vi "DCMotor_GetKrakenX44_FOC.vi"(11 "Num Motors":i32=1) -> (3 "DCMOTOR":T1 {"Jr_KgM2" format="%13.5p"; "L_H" format="%13.5p"; "Kt_NMPerAmp" format="%13.5p"; "KvINV_RadPerSecPerVolt" format="%13.5p"; "R_Ohms" format="%13.5p"; "FreeSpeed_RadPerSec" format="%13.5p"; "FreeCurrent_Amps" format="%13.5p"; "StallCurrent_Amps" format="%13.5p"; "StallTorque_NM" format="%13.5p"; "nominalVoltage_Volts" format="%13.5p"})   [LabVIEW 2019, in "Trajectory_Library.lvlib"]
doc: "Creates a new DC MOTOR data cluster with the specified values. for a set of Kraken X44 with FOC enabled motors. \n\nInputs: \n - Num Motors -- The number of motors used together in this sytem driving the same load.\n\nOutputs:\n - DCMOTOR -- Cluster containing the motor modeling constants for this set of motors."
uses:
  TypeDef/DCMOTOR.CTL
  Trajectory_Library.lvlib
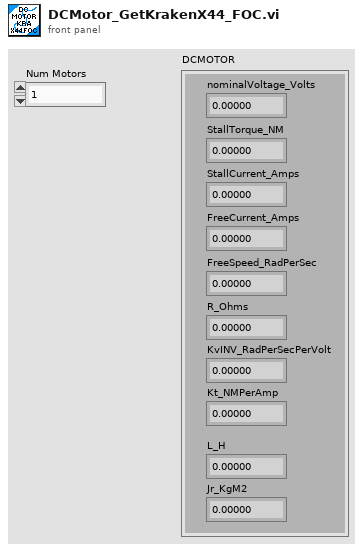
[diagram p1: front panel]
types:
  T1 = typedef "Trajectory_Library.lvlib/DCMOTOR.CTL" = cluster{"nominalVoltage_Volts":dbl, "StallTorque_NM":dbl, "StallCurrent_Amps":dbl, "FreeCurrent_Amps":dbl, "FreeSpeed_RadPerSec":dbl, "R_Ohms":dbl, "KvINV_RadPerSecPerVolt":dbl, "Kt_NMPerAmp":dbl, "L_H":dbl, "Jr_KgM2":dbl}
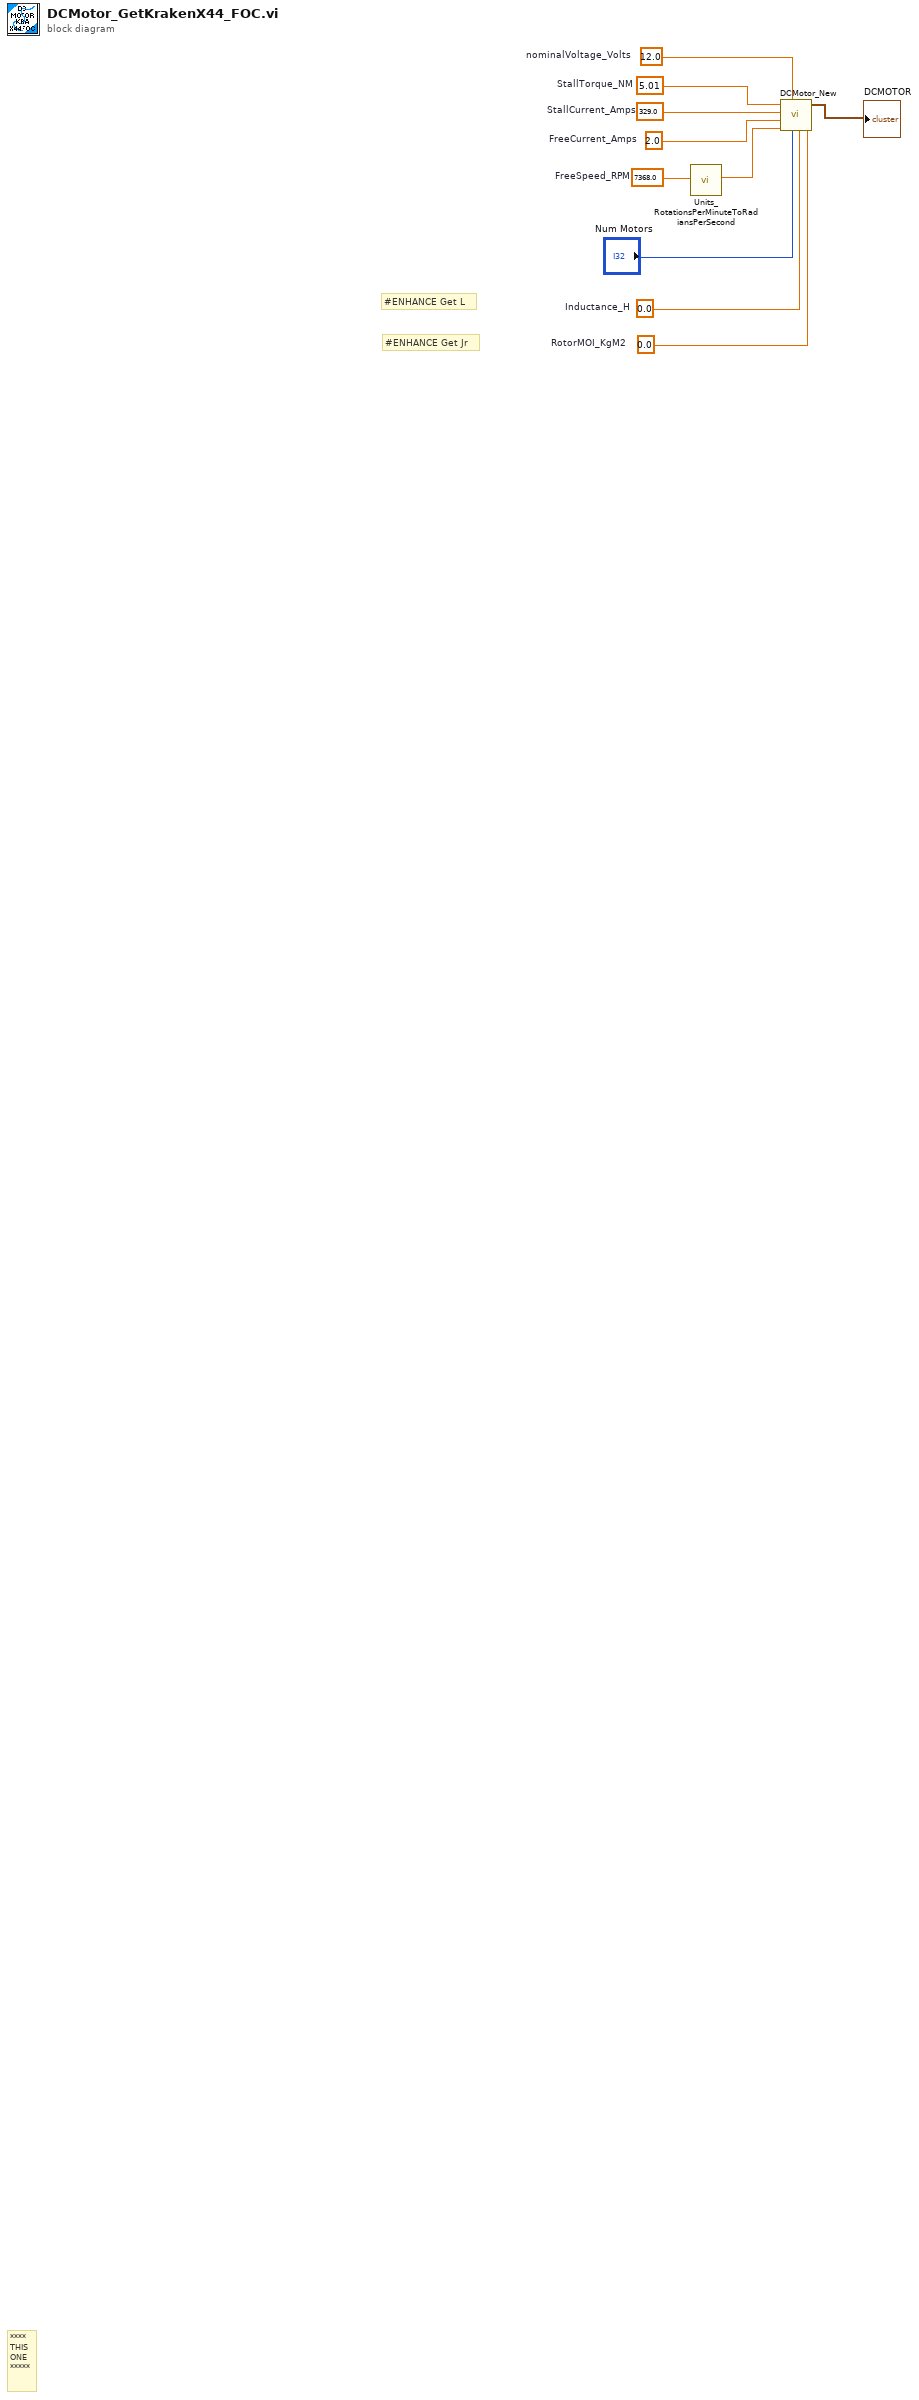
[diagram p0: block diagram]
diagram:
  w1 = 0.0  # RotorMOI_KgM2
  w2 = 0.0  # Inductance_H
  w4 = 7368.0  # FreeSpeed_RPM
  w5 = 2.0  # FreeCurrent_Amps
  w6 = 329.0  # StallCurrent_Amps
  w7 = 5.01  # StallTorque_NM
  w8 = 12.0  # nominalVoltage_Volts
  # "#ENHANCE Get L"
  # "#ENHANCE Get Jr"
  # "****\nTHIS\nONE\n*****"
  n1 = call "Units_RotationsPerMinuteToRadiansPerSecond.vi"("RotationsPerMinute"=w4) -> ("RadiansPerSecond"=w3:dbl)  [unwired: 10 in]
  n2 = call "DCMotor_New.vi"("RotorMOI_KgM2"=w1, "Inductance_H"=w2, "Num Motors"="Num Motors", "nominalVoltage_Volts"=w8, "FreeSpeed_RadPerSec"=w3, "FreeCurrent_Amps"=w5, "StallCurrent_Amps"=w6, "StallTorque_NM"=w7) -> ("DCMOTOR"=→"DCMOTOR":T1)  [unwired: 3 in]
